vi "Turn_screw.vi"(8 "Error In":errorcluster) -> (0 "Error Out":errorcluster)   [LabVIEW 2019]
uses:
  <vilib>/Platform/TimedLoop/XDataNode/timing_clust.ctl
  <vilib>/Platform/TimedLoop/XDataNode/nitl_modes.ctl
  <vilib>/Platform/TimedLoop/XDataNode/wakeup.ctl
  WSCbot_V3_Toolkit.lvlibp/WSCBOTV3_Toolkit/IO/LowLevel/IO_Chanel_DIO.ctl
  <vilib>/platform/TimedLoop/XDataNode/XDataNode.xnode
  WSCbot_V3_Toolkit.lvlibp
  <vilib>/Platform/TimedLoop/XDataNode/XDNodeRunTimeDep.lvlib
panel:
  out "Stop Output":bool
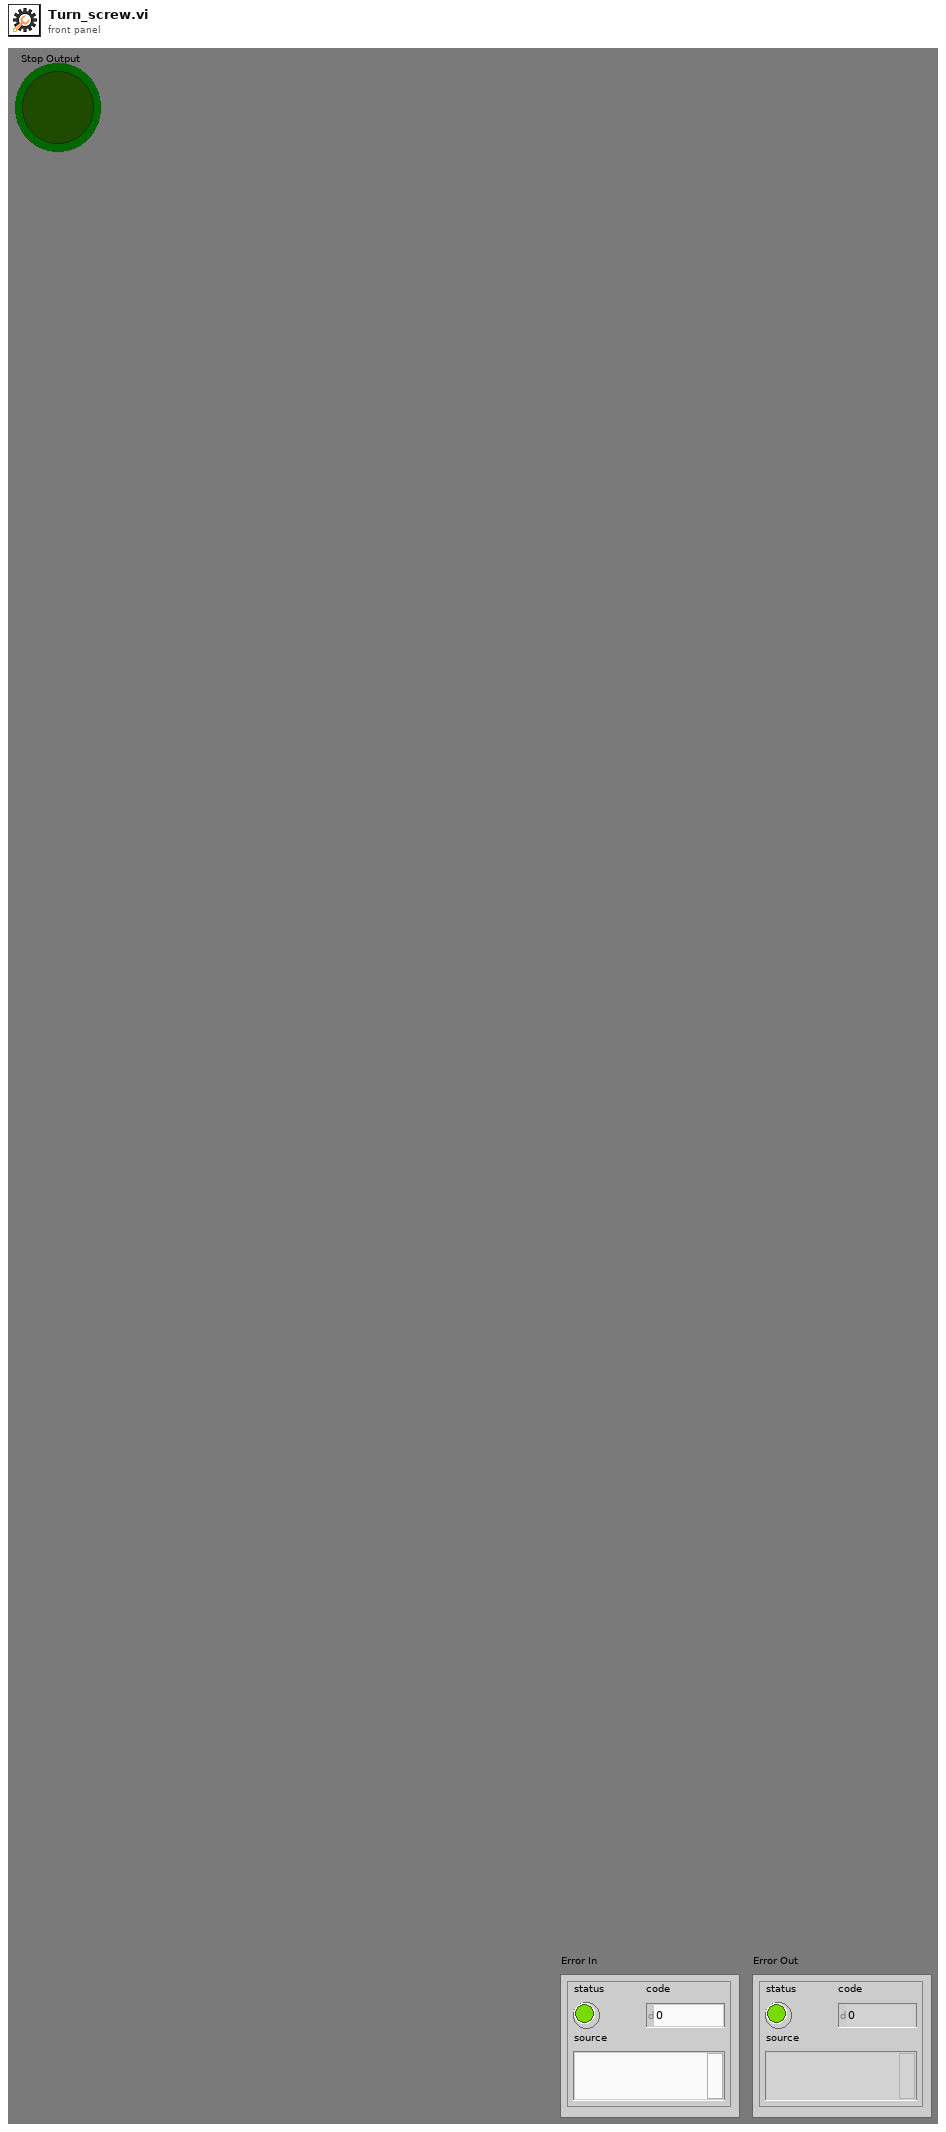
[diagram p1: front panel]
types:
  T1 = typedef "WSCbot_V3_Toolkit.lvlibp/IO_Chanel_DIO.ctl" = enum16{"A/DIO9", "A/DIO10", "C/DIO0", "C/DIO1", "C/DIO2", "C/DIO3", "C/DIO4", "C/DIO5", "C/DIO6"}
  T2 = typedef "XDNodeRunTimeDep.lvlib/timing_clust.ctl" = cluster{"Expected End [f-1]":u64, "Actual End [f-1]":u64, "Finished Late? [f-1]":bool, "Expected End [i-1]":u64, "Actual End [i-1]":u64, "Finished Late? [i-1]":bool, "Expected Start [i]":u64, "Actual Start [i]":u64, "Expected Start [f]":u64, "Actual Start [f]":u64, "Source Name":string, "Structure Name":string, "Period":i64, "Deadline":i64, "Offset":i64, "Start":i64, "Priority":i32, "Timeout":i32, "Mode":T3, "Wakeup Reason":T4, "Error":errorcluster, "Source Type":string, "Secondary Source Type":string, "Global End Time":u64, "Global Start Time":u64, "Frame Duration":u64, "Iteration Duration":u64, "Assigned CPU":i32, "I/O Scan Engine Mode":u32}
  T3 = typedef "XDNodeRunTimeDep.lvlib/nitl_modes.ctl" = enum32{"No Change", "Process missed periods, maintain original phase", "Discard missed periods, maintain original phase", "Process missed periods, ignore original phase", "Discard missed periods, ignore original phase"}
  T4 = typedef "XDNodeRunTimeDep.lvlib/wakeup.ctl" = enum32{"Normal", "Aborted", "Asynchronous wakeup", "Timing source error", "Timed loop error", "Timeout"}
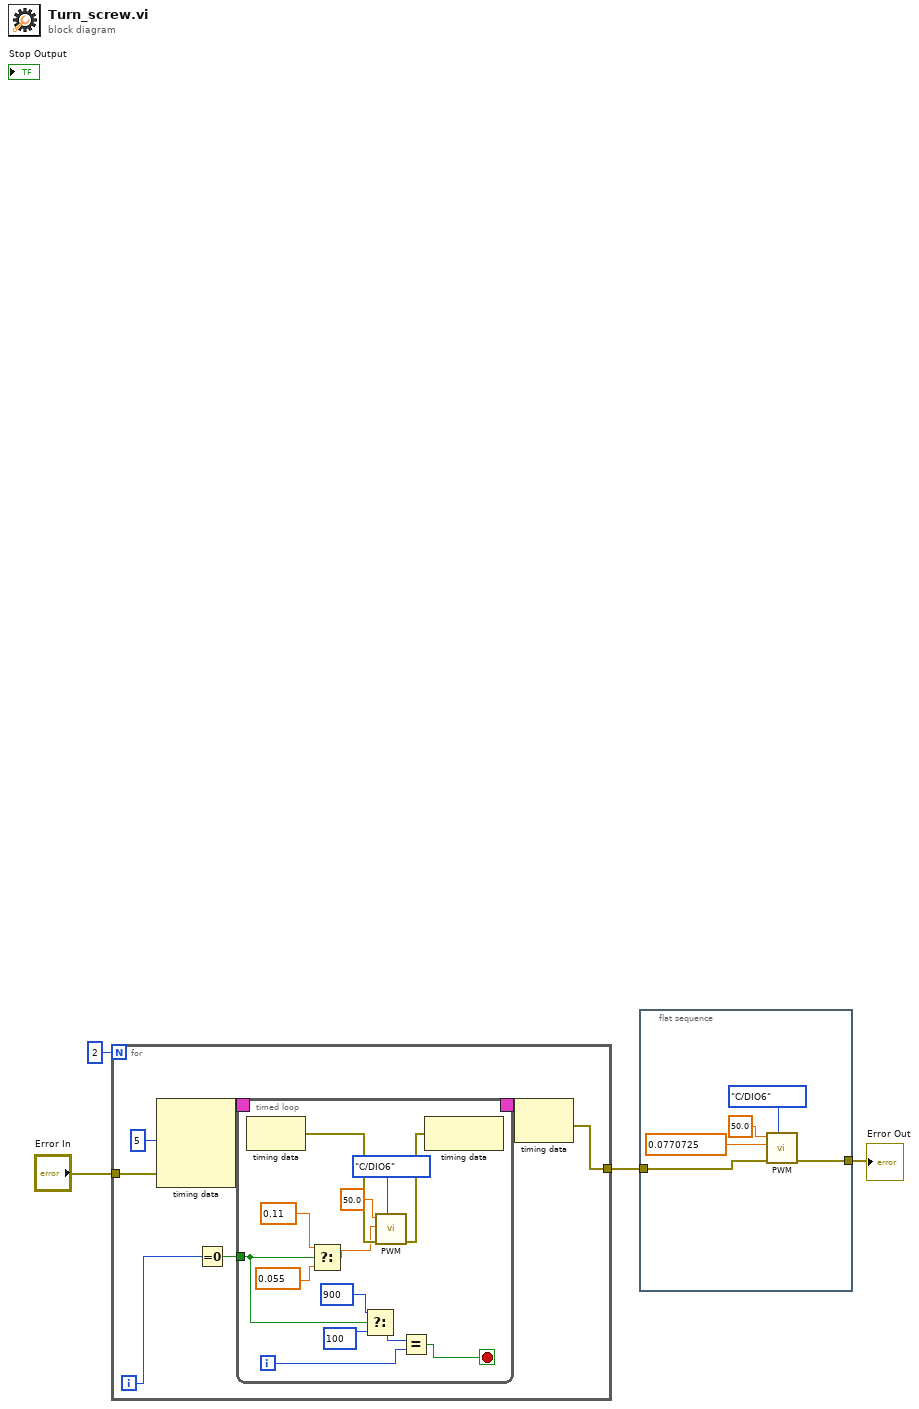
[diagram p0: block diagram]
diagram:
  n1 = for {
    N: 2 -> [_]
    tunnel: [w9] -> w1
    tunnel: "Error In" -> [w7]
    i -> [w6]
    n2 = node-c288(i64 5 ("Period"), w7) -> (w11:T2)  [unwired: 2 in]
    n3 = Equal To 0?(x=w6) -> (x = 0?=w5:bool)
    n4 = timed-loop {
      timing: w11 -> [_]
      timing-out: [_] -> w10
      tunnel: w5 -> [w15]
      i -> [w22]
      stop <- w12 stop-if-true
      n5 = node-c288() -> (w21:errorcluster)  [unwired: 1 in]
      n6 = Select(t=0.11 ("DutyCycle"), s=w15, f=0.055 ("DutyCycle")) -> (s? t:f=w18:dbl)
      n7 = Select(t=900 ("x"), s=w15, f=100) -> (s? t:f=w13:i32)
      n8 = call "PWM.vi"("IO_Chanel"=IO_Chanel_DIO."C/DIO6", "error in"=w21, "DutyCycle"=w18, "Frequency(Hz)"=50.0) -> ("error out"=w20:errorcluster)  [unwired: 7 in]
      n9 = Equal?(x=w13, y=w22) -> (x = y?=w12:bool)
      n10 = node-c288(w20) -> ()  [unwired: 1 out]
    }
    n11 = node-c288(w10) -> (w9:errorcluster)
  }
  n12 = flat-sequence {
    tunnel: [w37] -> w3
    tunnel: w1 -> [w36]
    frame #0 {
      n13 = call "PWM.vi"("IO_Chanel"=IO_Chanel_DIO."C/DIO6", "error in"=w36, "DutyCycle"=0.0770725, "Frequency(Hz)"=50.0) -> ("error out"=w37:errorcluster)  [unwired: 7 in]
    }
  }
  "Error Out" <- w3
